vi "Notifier_Driver.vi"(0 "Notification":bool, 2 "Notifier_Name":string, 11 "Error_In":errorcluster, 13 "Notifier_Operation_Select":T1=enum."Release_Notifier") -> (4 "Latest_Notification":bool, 15 "Error_Out":errorcluster)   [LabVIEW 2023]
uses:
  Controls/Notifier_Operation_Select.ctl
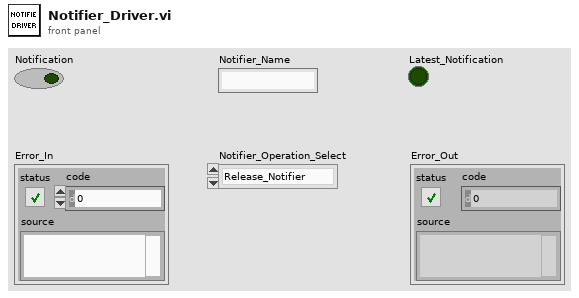
[diagram p1: front panel]
types:
  T1 = typedef "Notifier_Operation_Select.ctl" = enum16{"Obtain_Notifier", "Send_Notification", "Get_Notification_Status", "Release_Notifier"}
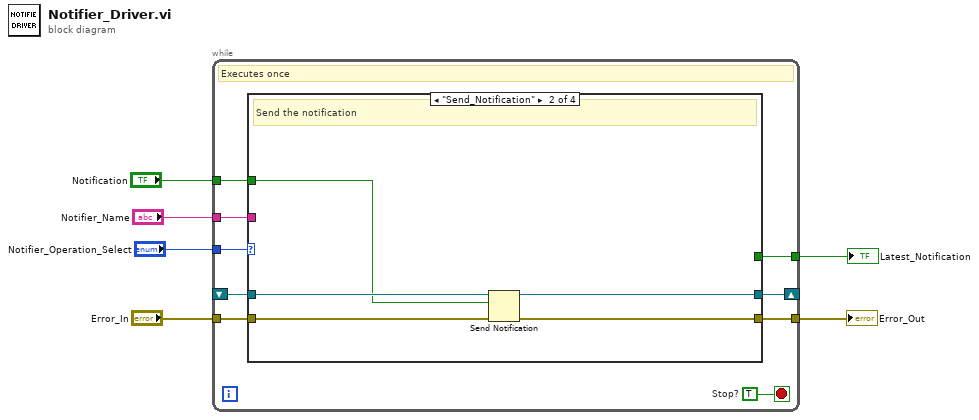
[diagram p0: block diagram]
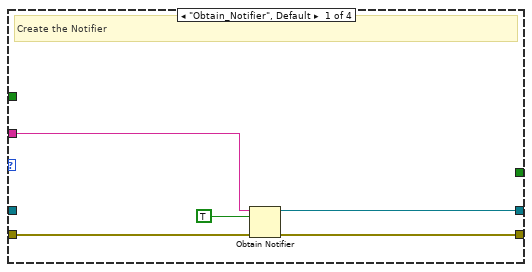
[diagram p2: hidden frame]
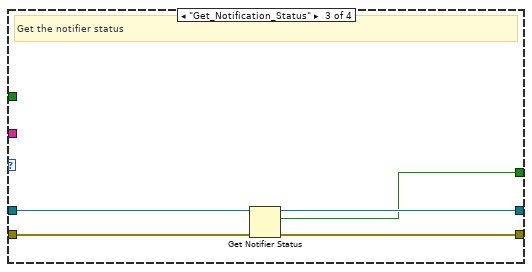
[diagram p3: hidden frame]
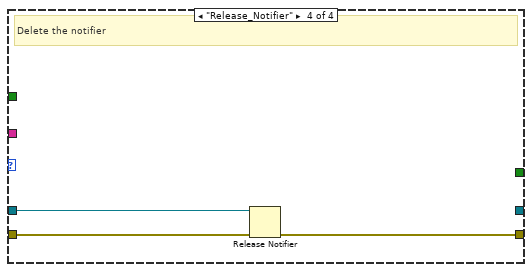
[diagram p4: hidden frame]
diagram:
  n1 = while {
    tunnel: "Notifier_Operation_Select" -> [w15]
    tunnel: "Error_In" -> [w14]
    tunnel: [w13] -> w4
    shift-right: [w12] -> _
    shift-left: _ -> [w11]
    tunnel: "Notifier_Name" -> [w10]
    tunnel: [w9] -> w2
    tunnel: "Notification" -> [w7]
    stop <- w8 stop-if-true
    w8 = TRUE  # Stop?
    # "Executes once"
    n2 = case shown="\"Send_Notification\"" w15 {
      tunnel: w14 -> [w20 w25 w30 w33]
      tunnel: [w19 w24 w29 w32] -> w13
      tunnel: [w16 w23 w27 _] -> w12
      tunnel: w11 -> [_ w22 w28 w31]
      tunnel: w10 -> [w18 _ _ _]
      tunnel: [_ _ w26 _] -> w9
      tunnel: w7 -> [_ w21 _ _]
      frame "Obtain_Notifier", Default {
        # "Create the Notifier"
        n3 = Obtain Notifier(name (unnamed)=w18, notification data type=TRUE, error in (no error)=w20) -> (notifier out=w16:refnum<notifier>, error out=w19:errorcluster)  [unwired: 1 in, 1 out]
      }
      frame "Send_Notification" {
        # "Send the notification"
        n4 = Send Notification(notification=w21, notifier=w22, error in (no error)=w25) -> (notifier out=w23:refnum<notifier>, error out=w24:errorcluster)
      }
      frame "Get_Notification_Status" {
        # "Get the notifier status"
        n5 = Get Notifier Status(notifier=w28, error in (no error)=w30) -> (notifier out=w27:refnum<notifier>, current notification=w26:bool, error out=w29:errorcluster)  [unwired: 2 out]
      }
      frame "Release_Notifier" {
        # "Delete the notifier"
        n6 = Release Notifier(notifier=w31, error in (no error)=w33) -> (error out=w32:errorcluster)  [unwired: 1 in, 2 out]
      }
    }
  }
  "Error_Out" <- w4
  "Latest_Notification" <- w2
